vi "Catagory Counts String.vi"(8 "error in (no error)":errorcluster {"code" format="Error %.0f"}, 11 "VIDoc Parser In":refnum<class "VIDoc Parser.lvclass">) -> (0 "error out":errorcluster {"code" format="Error %.0f"}, 2 "Catagory Counts":string, 3 "VIDoc Parser Out":refnum<class "VIDoc Parser.lvclass">)   [LabVIEW 2023, in "VIDoc Parsing.lvlib" / "VIDoc Parser.lvclass"]
uses:
  VIDoc Parser.lvclass
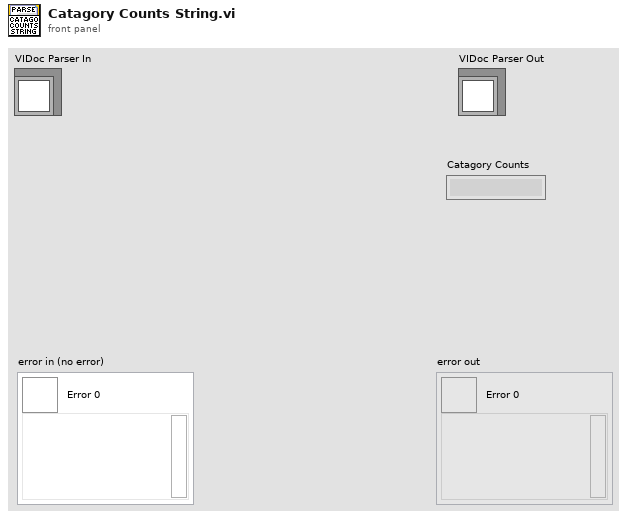
[diagram p1: front panel]
types:
  T1 = map{string, refnum<class "GUI Documentation.lvclass">[]}
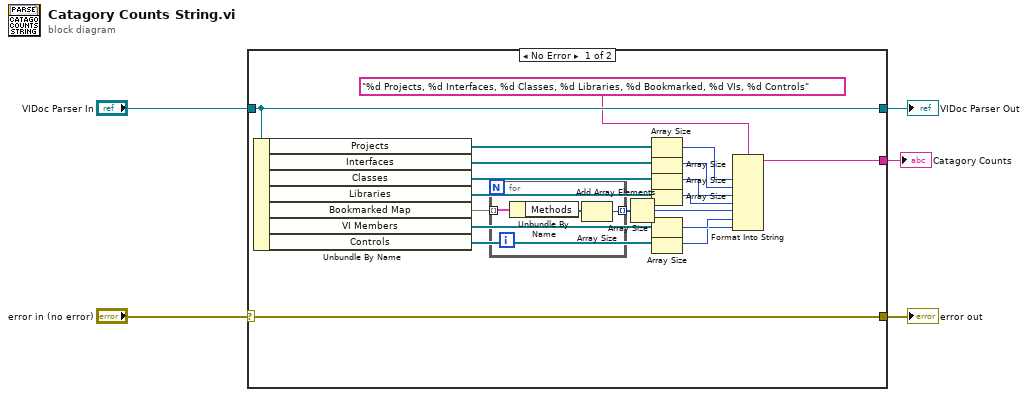
[diagram p0: block diagram]
diagram:
  n1 = case shown="No Error" "error in (no error)" {
    selector: "error in (no error)" -> [w24 w29]
    tunnel: [w24 w29] -> w4
    tunnel: [w23 w28] -> w2
    tunnel: "VIDoc Parser In" -> [w23 w28]
    tunnel: [w9 _] -> w1
    frame No Error {
      n2 = Unbundle By Name(w23) -> ("Projects"=w22:refnum<class "Project Documentation.lvclass">[], "Interfaces"=w21:refnum<class "Interface Documenation.lvclass">[], "Classes"=w20:refnum<class "Class Documentation.lvclass">[], "Libraries"=w19:refnum<class "Library Documentation.lvclass">[], "Bookmarked Map"=w8:T1, "VI Members"=w18:refnum<class "GUI Documentation.lvclass">[], "Controls"=w17:refnum<class "GUI Documentation.lvclass">[])
      n3 = for {
        tunnel: w8 -> [w27] mode=indexing
        tunnel: [w26] -> w7 mode=indexing
        n4 = Unbundle By Name(w27) -> ("Methods"=w25:refnum<class "GUI Documentation.lvclass">[])
        n5 = Array Size(array=w25) -> (size(s)=w26:i32)
      }
      n6 = Add Array Elements(numeric array=w7) -> (sum=w6:i32)
      n7 = Array Size(array=w22) -> (size(s)=w10:i32)
      n8 = Array Size(array=w21) -> (size(s)=w12:i32)
      n9 = Array Size(array=w20) -> (size(s)=w14:i32)
      n10 = Array Size(array=w19) -> (size(s)=w15:i32)
      n11 = Array Size(array=w18) -> (size(s)=w13:i32)
      n12 = Array Size(array=w17) -> (size(s)=w11:i32)
      n13 = Format Into String(format string="%d Projects, %d Interfaces, %d Classes, %d Libraries, %d Bookmarked, %d VIs, %d Controls", w10, w12, w14, w15, w6, w13, w11) -> (resulting string=w9:string)  [unwired: 2 in, 1 out]
    }
    frame Error {
    }
  }
  "error out" <- w4
  "VIDoc Parser Out" <- w2
  "Catagory Counts" <- w1
